vi "Common_Extra_Chs.vi"() -> (0 "Common Extra Channels":string[](array[string]))   [LabVIEW 2011]
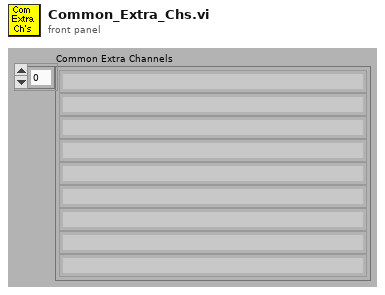
[diagram p1: front panel]
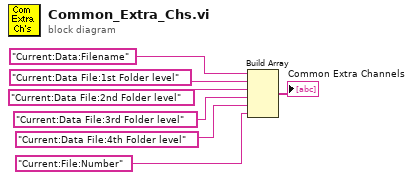
[diagram p0: block diagram]
diagram:
  n1 = Build Array("Current:Data:Filename", "Current:Data File:1st Folder level", "Current:Data File:2nd Folder level", "Current:Data File:3rd Folder level", "Current:Data File:4th Folder level", "Current:File:Number") -> (→"Common Extra Channels":string[])
